vi "cam.vi"() -> ()   [LabVIEW 2013]
uses:
  <vilib>/userdefined/High Color/IMAQdx.ctl
  <vilib>/vision/Image Controls.llb/IMAQ Image.ctl
  <vilib>/vision/driver/NI_Vision_Acquisition_Software.lvlib
panel:
  out "Rec Status":bool
  out "# elements in queue":i32
  in  "Image Path":path=path "C:/test"
  in  "Readme Path":path=path "C:/test/testreadme.txt"
  in  "Camera":T1="cam0"
  in  "REC":bool
  out "REC Image":T2(plugin-control)
  out "Image":T2(plugin-control)
  in  "stop":bool
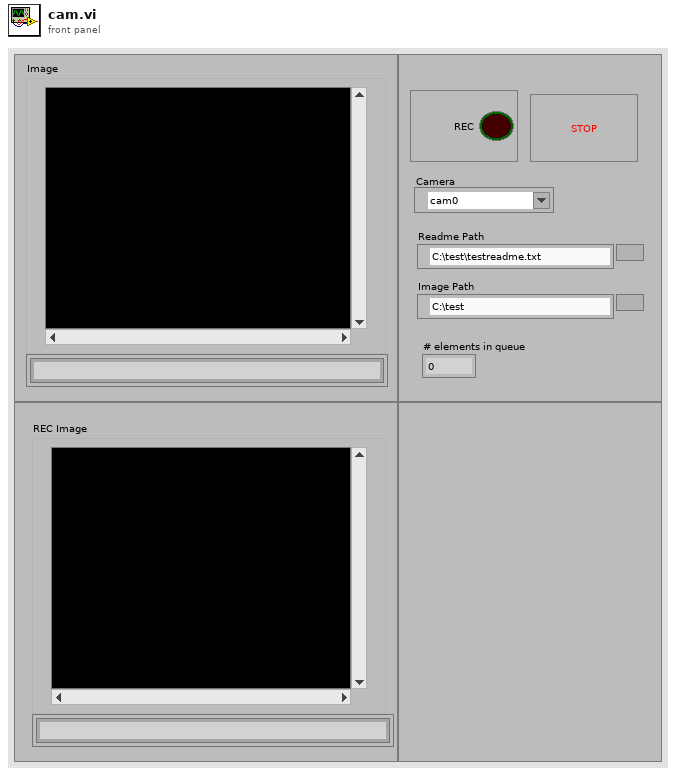
[diagram p1: front panel]
types:
  T1 = typedef "IMAQdx.ctl" = refnum<k21>
  T2 = typedef "IMAQ Image.ctl" = refnum<image>
  T3 = enum16{"open", "replace", "create", "open or create", "replace or create", "replace or create with confirmation"}
  T4 = cluster{"Image Out":T2, "seconds since 1Jan1904":timestamp}
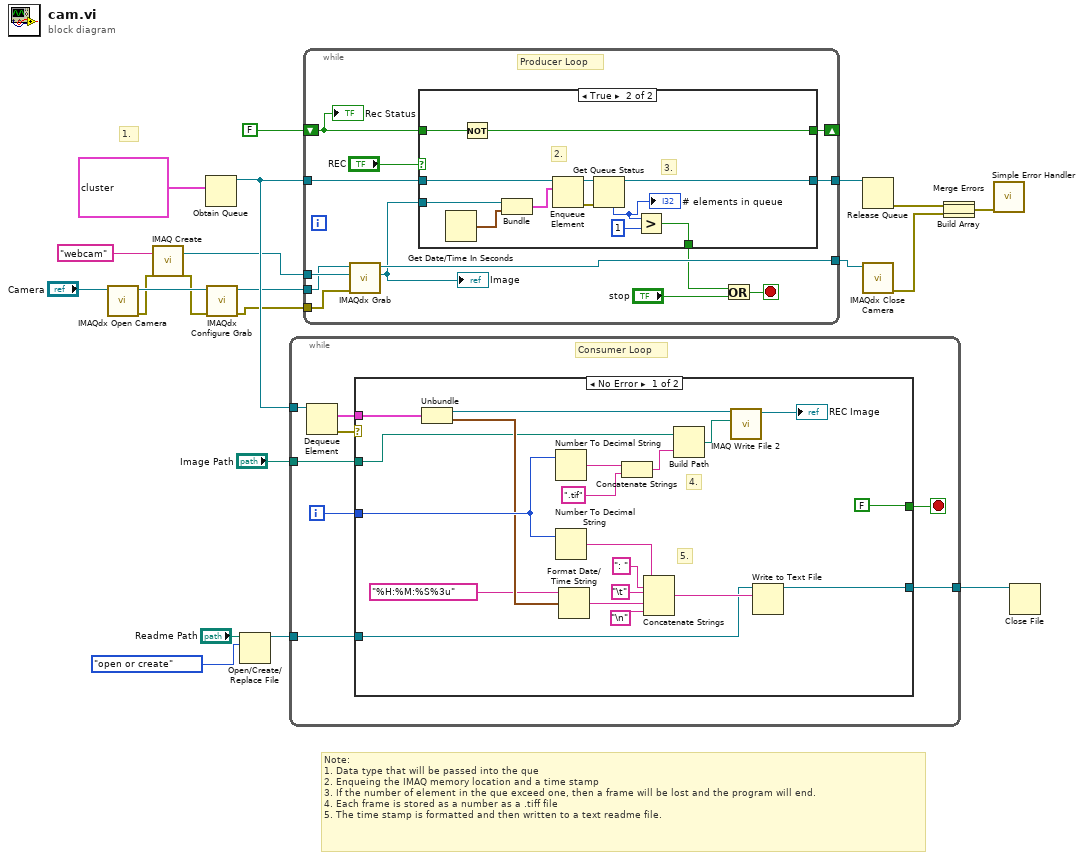
[diagram p0: block diagram]
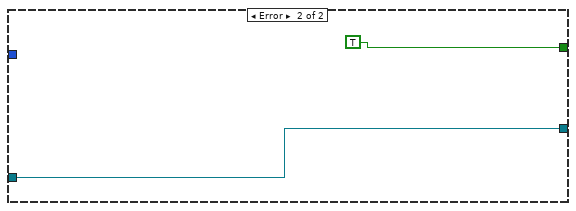
[diagram p2: hidden frame]
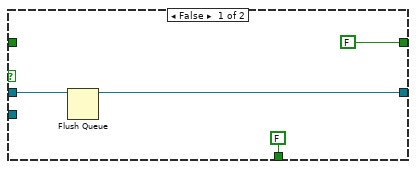
[diagram p3: hidden frame]
diagram:
  # "1."
  # "Note:\n1. Data type that will be passed into the que\n2. Enqueing the IMAQ memory location and a time stamp\n3. If the number of element in the que exceed one, then a frame will be lost and the program will end. \n4. Each frame is stored as a number as a .tiff file\n5. The time stamp is formatted and then written to a text readme file."
  n1 = call <vilib>:"IMAQdx Open Camera.vi"("Session In"="Camera") -> ("error out"=w5:errorcluster, "Session Out"=w20:T1)  [unwired: 9 in]
  n2 = call "IMAQ Create"("Image Name"="webcam", "error in (no error)"=w5) -> ("New Image"=w15:T2, "error out"=w4:errorcluster)  [unwired: 3 in]
  n3 = Obtain Queue(element data type=cluster{"Image":T2, "current time":timestamp} {"Image"="Webcam", "current time"=timestamp(0 s since 1904-01-01)}) -> (queue out=w22:refnum<queue>)  [unwired: 4 in, 2 out]
  n4 = call <vilib>:"IMAQdx Configure Grab.vi"("error in"=w4, "Session In"=w20) -> ("error out"=w3:errorcluster, "Session Out"=w17:T1)  [unwired: 8 in]
  n5 = Open/Create/Replace File(file path (use dialog)="Readme Path", operation (0:open)=T3."open or create") -> (refnum out=w9:refnum<file>)  [unwired: 4 in, 2 out]
  n6 = while {
    tunnel: w22 -> [w30]
    tunnel: [w25] -> w10
    tunnel: w9 -> [w24]
    tunnel: "Image Path" -> [w23]
    i -> [w26]
    stop <- w28 stop-if-true
    # "Consumer Loop"
    n7 = Dequeue Element(queue=w30) -> (element=w27:cluster{"Image":T2, "current time":timestamp}, error out=w29:errorcluster)  [unwired: 2 in, 2 out]
    n8 = case shown="No Error" w29 {
      tunnel: [FALSE TRUE] -> w28
      tunnel: w27 -> [w44 _]
      tunnel: w26 -> [w42 _]
      tunnel: [w41 w51] -> w25
      tunnel: w24 -> [w39 w51]
      tunnel: w23 -> [w31 _]
      frame No Error {
        # "5."
        # "4."
        n9 = Unbundle(w44) -> ("Image"=w43:T2, "current time"=w37:timestamp)
        n10 = Number To Decimal String(number=w42) -> (decimal integer string=w47:string)  [unwired: 1 in]
        n11 = Number To Decimal String(number=w42) -> (decimal integer string=w35:string)  [unwired: 1 in]
        n12 = Format Date/Time String(time format string (%c)="%H:%M:%S%3u", seconds (now)=w37) -> (date/time string=w36:string)  [unwired: 1 in]
        n13 = Concatenate Strings(w47, ".tif" ("string")) -> (w45:string)
        n14 = Concatenate Strings(w35, ": " ("string"), "\t", w36, "\n") -> (w40:string)
        n15 = Build Path(base path=w31, name or relative path=w45) -> (appended path=w48:path)
        n16 = call-poly "IMAQ Write File 2"("File Path"=w48, "Image"=w43) -> ("Image Out (duplicate)"=→"REC Image":T2)  [unwired: 8 in, 1 out]
        n17 = Write to Text File(file (use dialog)=w39, text=w40) -> (refnum out=w41:refnum<file>)  [unwired: 2 in, 2 out]
      }
      frame Error {
      }
    }
  }
  n18 = while {
    tunnel: w22 -> [w65]
    tunnel: [w64] -> w21
    tunnel: w15 -> [w63]
    tunnel: w17 -> [w62]
    tunnel: [w61] -> w16
    tunnel: w3 -> [w55]
    shift-right: [w53] -> _
    shift-left: FALSE -> [w54]
    stop <- w56 stop-if-true
    # "Producer Loop"
    n19 = call <vilib>:"IMAQdx Grab.vi"("error in"=w55, "Image In"=w63, "Session In"=w62) -> ("Image Out"=w60:T2, "Session Out"=w61:T1)  [unwired: 5 in, 2 out]
    "Image" <- w60
    n20 = case shown="True" "REC" {
      tunnel: w65 -> [w69 w81]
      tunnel: [w68 w76] -> w64
      tunnel: w60 -> [_ w79]
      tunnel: [FALSE w74] -> w58
      tunnel: w54 -> [_ w71]
      tunnel: [FALSE w70] -> w53
      frame False {
        n21 = Flush Queue(queue=w69) -> (queue out=w68:refnum<queue>)  [unwired: 1 in, 2 out]
      }
      frame True {
        # "3."
        # "2."
        n22 = Get Date/Time In Seconds() -> (seconds since 1Jan1904=w80:timestamp)
        n23 = Not(x=w71) -> (.not. x?=w70:bool)
        n24 = Bundle("Image Out"=w79, "seconds since 1Jan1904"=w80) -> (w78:T4)  [unwired: 1 in]
        n25 = Enqueue Element(queue=w81, element=w78) -> (queue out=w77:refnum<queue>, error out=w73:errorcluster)  [unwired: 2 in, 1 out]
        n26 = Get Queue Status(queue=w77, error in (no error)=w73) -> (queue out=w76:refnum<queue>, # elements in queue=w72:i32)  [unwired: 1 in, 6 out]
        "# elements in queue" <- w72
        n27 = Greater?(x=w72, y=1) -> (0:w74:bool)
      }
    }
    n28 = Or(x=w58, y="stop") -> (x .or. y?=w56:bool)
    "Rec Status" <- w54
  }
  n29 = Release Queue(queue=w21) -> (error out=w14:errorcluster)  [unwired: 2 in, 2 out]
  n30 = call <vilib>:"IMAQdx Close Camera.vi"("Session In"=w16) -> ("error out"=w13:errorcluster)  [unwired: 10 in]
  n31 = Build Array(w14, w13) -> (w1:errorcluster[])
  n32 = Merge Errors(w1) -> (w12:errorcluster)
  n33 = call <vilib>:"Simple Error Handler.vi"("error in (no error)"=w12) -> ()  [unwired: 4 in, 5 out]
  n34 = Close File(refnum=w10) -> ()  [unwired: 1 in, 2 out]
